vi "FilterAndCloseSpecifiedReferences.vi"(6 "Control references to filter":refnum<vi>[](array[refnum]), 8 "error in (no error)":errorcluster, 10 "Control references to close":refnum<vi>[](array[refnum])) -> (0 "error out":errorcluster)   [LabVIEW 2017, in "ErrorStructureDrawer.lvlib"]
doc: "Close the specified control references, except for anything also specified in the filter"
uses:
  ErrorStructureDrawer.lvlib
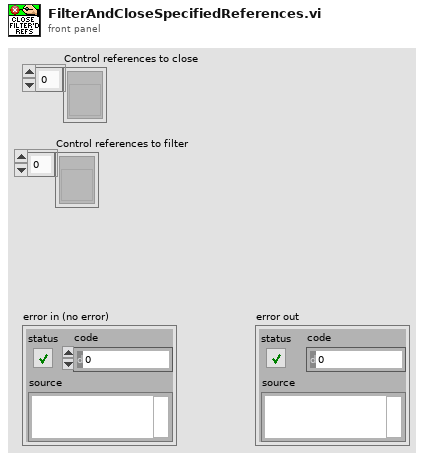
[diagram p1: front panel]
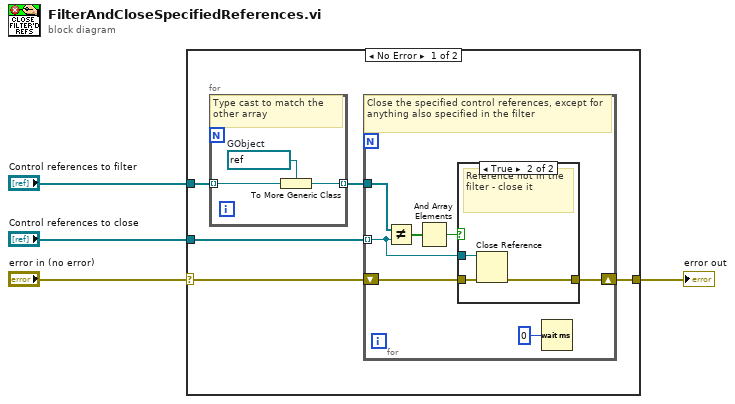
[diagram p0: block diagram]
diagram:
  n1 = case shown="No Error" "error in (no error)" {
    selector: "error in (no error)" -> [w7 w24]
    tunnel: [w9 w24] -> w4
    tunnel: "Control references to close" -> [w8 _]
    tunnel: "Control references to filter" -> [w6 _]
    frame No Error {
      n2 = for {
        tunnel: w6 -> [w12] mode=indexing
        tunnel: [w11] -> w5 mode=indexing
        w10 = refnum<vi> refnum  # GObject
        # "Type cast to match the other array"
        n3 = To More Generic Class(target class=w10, reference=w12) -> (generic class reference=w11:refnum<vi>)
      }
      n4 = for {
        tunnel: w8 -> [w15] mode=indexing
        shift-right: [w18] -> w9
        shift-left: w7 -> [w19]
        tunnel: w5 -> [w16]
        # "Close the specified control references, except for anything also specified in the filter"
        n5 = Not Equal?(x=w16, y=w15) -> (x != y?=w14:bool[])
        n6 = And Array Elements(Boolean array=w14) -> (logical AND=w13:bool)
        n7 = case shown="True" w13 {
          tunnel: w19 -> [w20 w23]
          tunnel: [w20 w22] -> w18
          tunnel: w15 -> [_ w21]
          frame False {
            # "Reference is in the filter - do nothing"
          }
          frame True {
            # "Reference not in the filter - close it"
            n8 = Close Reference(reference=w21, error in (no error)=w23) -> (error out=w22:errorcluster)
          }
        }
        n9 = Wait (ms)(milliseconds to wait=u32 0) -> ()  [unwired: 1 out]
      }
    }
    frame Error {
    }
  }
  "error out" <- w4
